vi "Configure Session.vi"(8 "error in":errorcluster, 11 "Plugin in":refnum<class "Configure Visa Device Channels.lvclass">) -> (0 "error out":errorcluster, 3 "Plugin out":refnum<class "Configure Visa Device Channels.lvclass">)   [LabVIEW 2026, in "Configure Visa Device Channels.lvlib" / "Configure Visa Device Channels.lvclass"]
uses:
  Configure Visa Device Channels.lvclass
  C:/Program Files/National Instruments/LabVIEW 2026/vi.lib/FlexLogger/SDK/PluginSDK.lvlibp/PEFClasses/SDK/Plugin/Plugin.lvclass
  Configure Visa Device Channels.lvclass/Configure Visa Device Channels.ctl
  <vilib>/FlexLogger/SDK/PluginSDK.lvlibp/PEFClasses/SDK/Plugin/ParameterAccess/Read String.vi
  <vilib>/FlexLogger/SDK/PluginSDK.lvlibp/PEFClasses/SDK/Plugin/ParameterAccess/Read I32.vi
  <vilib>/FlexLogger/SDK/PluginSDK.lvlibp/PEFClasses/SDK/Plugin/Plugin.lvclass
  C:/Program Files/National Instruments/LabVIEW 2026/vi.lib/FlexLogger/SDK/PluginSDK.lvlibp/PEFClasses/SDK/Processing Element/Processing Element.lvclass
  C:/Users/mpetrovi/OneDrive - Emerson/Documents/LabVIEW Projects/FlexLogger IO Plug-ins/Configure Visa Device Channels/Configure Visa Device Channels.lvclass
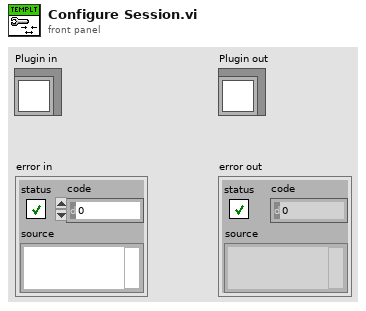
[diagram p1: front panel]
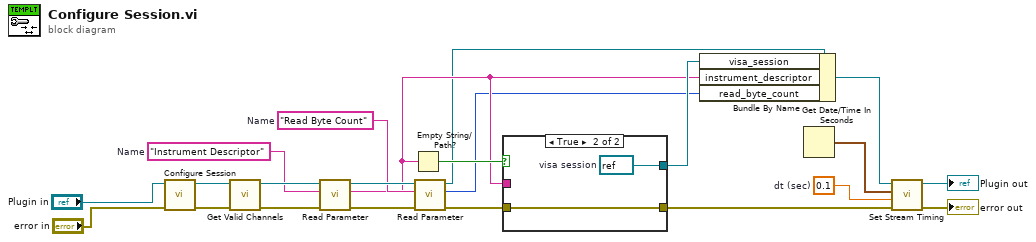
[diagram p0: block diagram]
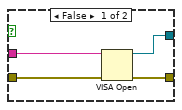
[diagram p2: hidden frame]
diagram:
  w4 = 0.1  # dt (sec)
  w14 = "Read Byte Count"  # Name
  w17 = "Instrument Descriptor"  # Name
  n1 = call-parent "Configure Session.vi"("error in (no error)"="error in", "Processing Element in"="Plugin in") -> ("error out"=w19:errorcluster, "Processing Element out"=w20:refnum<class "Configure Visa Device Channels.lvclass">)  [unwired: 8 in]
  n2 = call <vilib>:"Get Valid Channels.vi"("error in (no error)"=w19, "Plugin in"=w20) -> ("error out"=w16:errorcluster, "Plugin out"=w18:refnum<class "Configure Visa Device Channels.lvclass">)  [unwired: 7 in, 1 out]
  n3 = call-poly <vilib>:"Read Parameter.vi"("error in (no error)"=w16, "Name"=w17, "Plugin in"=w18) -> ("error out"=w13:errorcluster, "Value"=w9:string, "Plugin out"=w15:refnum<class "Configure Visa Device Channels.lvclass">)  [unwired: 5 in, 1 out]
  n4 = Empty String/Path?(string/path=w9) -> (empty?=w11:bool)
  n5 = call-poly <vilib>:"Read Parameter.vi"("error in (no error)"=w13, "Name"=w14, "Plugin in"=w15) -> ("error out"=w12:errorcluster, "Value"=w8:i32, "Plugin out"=w7:refnum<class "Configure Visa Device Channels.lvclass">)  [unwired: 5 in, 1 out]
  n6 = case shown="True" w11 {
    tunnel: w9 -> [w26 _]
    tunnel: w12 -> [w25 w27]
    tunnel: [w24 w28] -> w10
    tunnel: [w23 w27] -> w3
    frame False {
      n7 = VISA Open(error in (no error)=w25, VISA resource name=w26) -> (VISA resource name=w24:refnum<visa-resource-name>, error out=w23:errorcluster)  [unwired: 3 in]
    }
    frame True {
      w28 = refnum<visa-resource-name> refnum  # visa session
    }
  }
  n8 = Bundle By Name(cluster=w7, "visa_session"=w10, "instrument_descriptor"=w9, "read_byte_count"=w8) -> (w6:refnum<class "Configure Visa Device Channels.lvclass">)
  n9 = Get Date/Time In Seconds() -> (seconds since 1Jan1904=w5:timestamp)
  n10 = call-dynamic "Set Stream Timing.vi"("error in (no error)"=w3, "dt(sec)"=w4, "Start Time"=w5, "Plugin in"=w6) -> ("error out"=→"error out":errorcluster, "Plugin out"=→"Plugin out":refnum<class "Configure Visa Device Channels.lvclass">)  [unwired: 6 in]
